vi "hrdl (1).vi"() -> ()   [LabVIEW 2014]
uses:
  PicoHRDL.dll
panel:
  in  "milliseconds to wait":u32
  in  "stop":bool
  out "Waveform Chart":dbl(graph)
  out "Numeric":dbl
  out "Over Voltage":i16
  out "Handle":i16
  in  "Single Ended":i16 min=0 max=1 step=1
  in  "Conversion":i16 min=0 max=5 step=1
  in  "Voltage Range":i16 min=0 max=6 step=1
  in  "Channel":i16=1 min=1 max=16 step=1
  # "-1        if the unit fails to open\n0         if no unit is found\n>= 1   handle to the device opened"
  # "The channel that will be enabled or disabled.\nADC-20: 1 to 8\nADC-24: 1 to 16"
  # "Non-zero to measure a single-ended voltage.\nZero for a differential voltage."
  # "range Voltage range Availability\n (0)    ±2500 mV        ADC-20 and ADC-24\n (1)    ±1250 mV        ADC-20 and ADC-24\n (2)    ±625 mV          ADC-24 only\n (3)    ±312.5 mV       ADC-24 only\n (4)    ±156.25 mV     ADC-24 only\n (5)    ±78.125 mV     ADC-24 only\n (6)    ±39.0625 mV   ADC-24 only"
  # "conversion Conversion time\n(0)               60 ms\n(1)               100 ms\n(2)               180 ms\n(3)               340 ms\n(4)               660 ms"
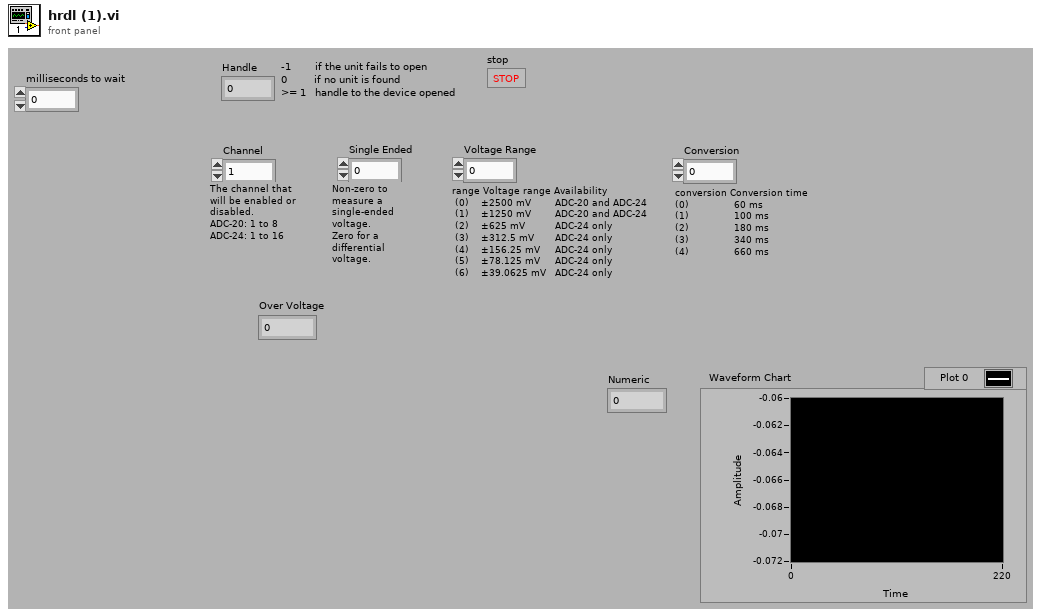
[diagram p1: front panel]
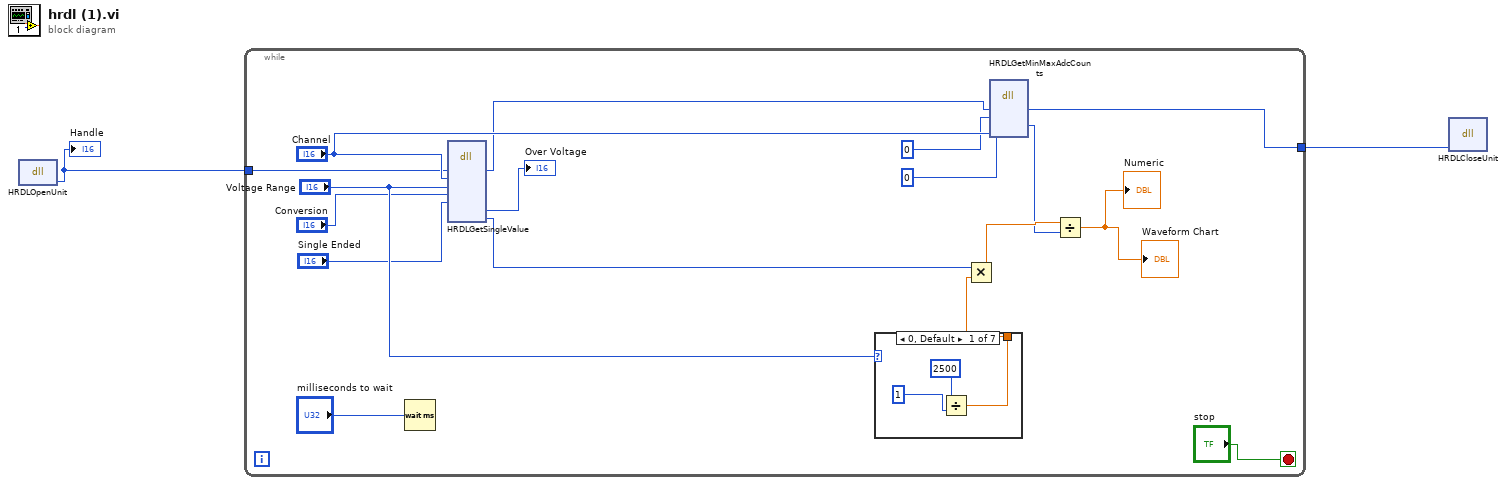
[diagram p0: block diagram]
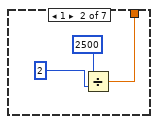
[diagram p2: hidden frame]
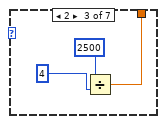
[diagram p3: hidden frame]
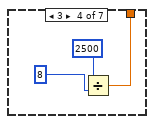
[diagram p4: hidden frame]
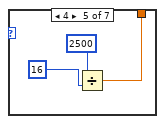
[diagram p5: hidden frame]
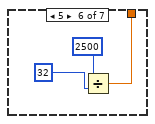
[diagram p6: hidden frame]
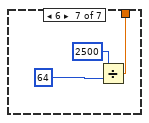
[diagram p7: hidden frame]
diagram:
  n1 = dll-call lib="PicoHRDL.dll" fn="HRDLOpenUnit"() -> ("return type"=w2:i16)  [unwired: 3 in, 2 out]
  "Handle" <- w2
  n2 = while {
    tunnel: w2 -> [w17]
    tunnel: [w6] -> w1
    stop <- "stop" stop-if-true
    n3 = Wait (ms)(milliseconds to wait="milliseconds to wait") -> ()  [unwired: 1 out]
    n4 = dll-call lib="PicoHRDL.dll" fn="HRDLGetSingleValue"("handle"=w17, "channel"="Channel", "range"="Voltage Range", "conversionTime"="Conversion", "singleEnded"="Single Ended") -> ("handle"=w7:i16, "overflow"=→"Over Voltage":i16, "value"=w4:i32)  [unwired: 10 in, 2 out]
    n5 = case shown="0, Default" "Voltage Range" {
      tunnel: [w20 w23 w26 w29 w32 w35 w38] -> w13
      frame 0, Default {
        n6 = Divide(x=2500, y=1) -> (x/y=w20:dbl)
      }
      frame 1 {
        n7 = Divide(x=2500, y=2) -> (x/y=w23:dbl)
      }
      frame 2 {
        n8 = Divide(x=2500, y=4) -> (x/y=w26:dbl)
      }
      frame 3 {
        n9 = Divide(x=2500, y=8) -> (x/y=w29:dbl)
      }
      frame 4 {
        n10 = Divide(x=2500, y=16) -> (x/y=w32:dbl)
      }
      frame 5 {
        n11 = Divide(x=2500, y=32) -> (x/y=w35:dbl)
      }
      frame 6 {
        n12 = Divide(x=2500, y=64) -> (x/y=w38:dbl)
      }
    }
    n13 = Multiply(x=w4, y=w13) -> (x*y=w12:dbl)
    n14 = dll-call lib="PicoHRDL.dll" fn="HRDLGetMinMaxAdcCounts"("handle"=w7, "minAdc"=0, "maxAdc"=0, "channel"="Channel") -> ("handle"=w6:i16, "maxAdc"=w11:i32)  [unwired: 6 in, 2 out]
    n15 = Divide(x=w12, y=w11) -> (x/y=→"Numeric" →"Waveform Chart":dbl)
  }
  n16 = dll-call lib="PicoHRDL.dll" fn="HRDLCloseUnit"("handle"=w1) -> ()  [unwired: 5 in, 2 out]
